vi "PulseDetect80AndSwitch160_10_HostTest.vi"(6 "Switch for":i32=6, 8 "Fill from last":i32=6, 9 "Laser bits in":bool[](array[boolean])=[FALSE, FALSE, FALSE, FALSE, FALSE, FALSE, FALSE, FALSE, FALSE, FALSE], 10 "Last area in":bool=TRUE, 11 "Last laser bit in":bool) -> (0 "Fill after last":i32=6, 1 "Area array out":bool[](array[boolean]), 2 "New last area out":bool, 3 "New last laser bit out":bool)   [LabVIEW 2012]
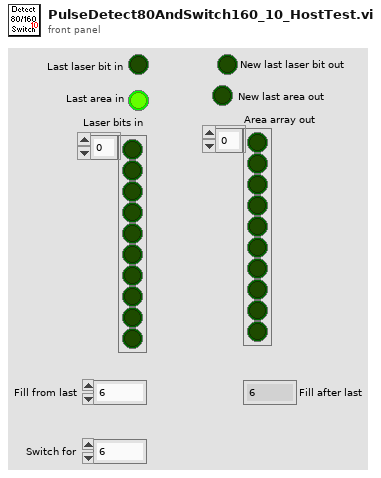
[diagram p1: front panel]
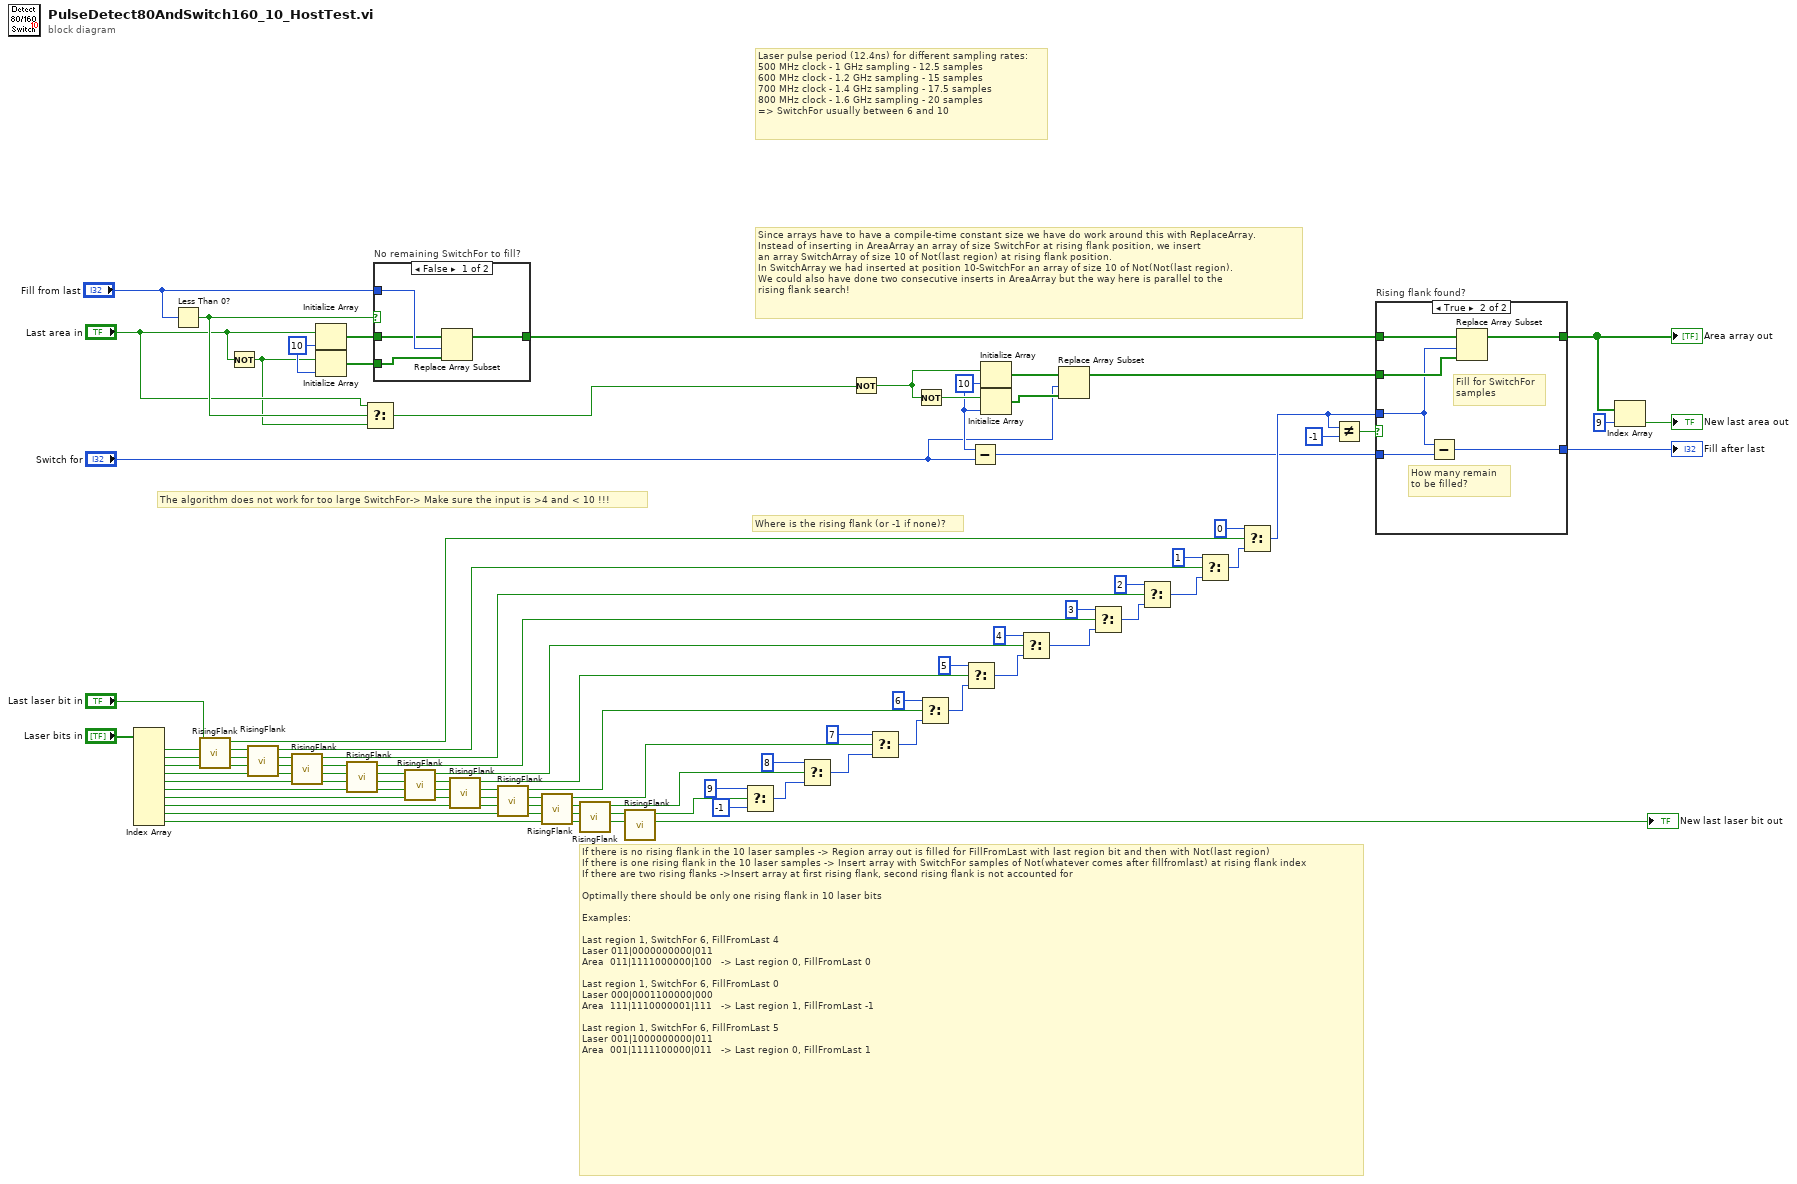
[diagram p0: block diagram]
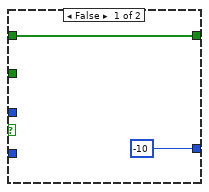
[diagram p3: hidden frame]
diagram:
  w7 = 10 ("dimension size")
  w15 = 10 ("dimension size")
  # "Since arrays have to have a compile-time constant size we have do work around this with ReplaceArray.\nInstead of inserting in AreaArray an array of size SwitchFor at rising flank position, we insert \nan array SwitchArray of size 10 of Not(last region) at rising flank position.\nIn SwitchArray we had inserted at position 10-SwitchFor an array of size 10 of Not(Not(last region).\nWe could also have done two consecutive inserts in AreaArray but the way here is parallel to the \nrising flank search!"
  # "The algorithm does not work for too large SwitchFor-> Make sure the input is >4 and < 10 !!!"
  # "Where is the rising flank (or -1 if none)?"
  # "Laser pulse period (12.4ns) for different sampling rates:\n500 MHz clock - 1 GHz sampling - 12.5 samples\n600 MHz clock - 1.2 GHz sampling - 15 samples\n700 MHz clock - 1.4 GHz sampling - 17.5 samples\n800 MHz clock - 1.6 GHz sampling - 20 samples \n=> SwitchFor usually between 6 and 10"
  # "If there is no rising flank in the 10 laser samples -> Region array out is filled for FillFromLast with last region bit and then with Not(last region)\nIf there is one rising flank in the 10 laser samples -> Insert array with SwitchFor samples of Not(whatever comes after fillfromlast) at rising flank index\nIf there are two rising flanks ->Insert array at first rising flank, second rising flank is not accounted for\n\nOptimally there should be only one rising flank in 10 laser bits\n\nExamples:\n\nLast region 1, SwitchFor 6, FillFromLast 4\nLaser 011|0000000000|011\nArea  011|1111000000|100   -> Last region 0, FillFromLast 0\n\nLast region 1, SwitchFor 6, FillFromLast 0\nLaser 000|0001100000|000\nArea  111|1110000001|111   -> Last region 1, FillFromLast -1\n\nLast region 1, SwitchFor 6, FillFromLast 5\nLaser 001|1000000000|011\nArea  001|1111100000|011   -> Last region 0, FillFromLast 1"
  n1 = Index Array(array="Laser bits in") -> (element #1=w64:bool, element #2=w63:bool, element #3=w62:bool, element #4=w61:bool, element #5=w60:bool, element #6=w59:bool, element #7=w58:bool, element #8=w57:bool, element #9=w56:bool, element #10=w38:bool)  [unwired: 10 in]
  "New last laser bit out" <- w38
  n2 = Less Than 0?(x="Fill from last") -> (x < 0?=w4:bool)
  n3 = call "RisingFlank.vi"("2nd sample"=w64, "1st sample"="Last laser bit in") -> ("Rising flank?"=w55:bool)  [unwired: 7 in]
  n4 = Not(x="Last area in") -> (.not. x?=w2:bool)
  n5 = call "RisingFlank.vi"("2nd sample"=w63, "1st sample"=w64) -> ("Rising flank?"=w53:bool)  [unwired: 7 in]
  n6 = call "RisingFlank.vi"("2nd sample"=w62, "1st sample"=w63) -> ("Rising flank?"=w51:bool)  [unwired: 7 in]
  n7 = Initialize Array("Last area in", w15) -> (w16:bool[])
  n8 = Initialize Array(w2, w15) -> (w14:bool[])
  n9 = call "RisingFlank.vi"("2nd sample"=w61, "1st sample"=w62) -> ("Rising flank?"=w36:bool)  [unwired: 7 in]
  n10 = Select(t="Last area in", s=w4, f=w2) -> (s? t:f=w1:bool)
  n11 = case "No remaining SwitchFor to fill?" shown="False" w4 {
    tunnel: [w67 w71] -> w13
    tunnel: "Fill from last" -> [w70 _]
    tunnel: w16 -> [w69 w71]
    tunnel: w14 -> [w68 _]
    frame False {
      n12 = Replace Array Subset(array=w69, new element=w68, index=w70) -> (w67:bool[])
    }
    frame True {
    }
  }
  n13 = call "RisingFlank.vi"("2nd sample"=w60, "1st sample"=w61) -> ("Rising flank?"=w49:bool)  [unwired: 7 in]
  n14 = call "RisingFlank.vi"("2nd sample"=w59, "1st sample"=w60) -> ("Rising flank?"=w47:bool)  [unwired: 7 in]
  n15 = call "RisingFlank.vi"("2nd sample"=w58, "1st sample"=w59) -> ("Rising flank?"=w45:bool)  [unwired: 7 in]
  n16 = call "RisingFlank.vi"("2nd sample"=w57, "1st sample"=w58) -> ("Rising flank?"=w43:bool)  [unwired: 7 in]
  n17 = call "RisingFlank.vi"("2nd sample"=w56, "1st sample"=w57) -> ("Rising flank?"=w41:bool)  [unwired: 7 in]
  n18 = call "RisingFlank.vi"("2nd sample"=w38, "1st sample"=w56) -> ("Rising flank?"=w39:bool)  [unwired: 7 in]
  n19 = Select(t=9, s=w39, f=-1) -> (s? t:f=w28:i32)
  n20 = Select(t=8, s=w41, f=w28) -> (s? t:f=w27:i32)
  n21 = Not(x=w1) -> (.not. x?=w11:bool)
  n22 = Select(t=7, s=w43, f=w27) -> (s? t:f=w26:i32)
  n23 = Not(x=w11) -> (.not. x?=w9:bool)
  n24 = Select(t=6, s=w45, f=w26) -> (s? t:f=w25:i32)
  n25 = Select(t=5, s=w47, f=w25) -> (s? t:f=w24:i32)
  n26 = Subtract(x=w7, y="Switch for") -> (x-y=w6:i32)
  n27 = Initialize Array(w11, w7) -> (w12:bool[])
  n28 = Initialize Array(w9, w7) -> (w8:bool[])
  n29 = Select(t=4, s=w49, f=w24) -> (s? t:f=w23:i32)
  n30 = Replace Array Subset(array=w12, new element=w8, index="Switch for") -> (w10:bool[])
  n31 = Select(t=3, s=w36, f=w23) -> (s? t:f=w22:i32)
  n32 = Select(t=2, s=w51, f=w22) -> (s? t:f=w21:i32)
  n33 = Select(t=1, s=w53, f=w21) -> (s? t:f=w20:i32)
  n34 = Select(t=0, s=w55, f=w20) -> (s? t:f=w19:i32)
  n35 = Not Equal?(x=w19, y=-1) -> (x != y?=w34:bool)
  n36 = case "Rising flank found?" shown="True" w34 {
    tunnel: w13 -> [w73 w79]
    tunnel: w10 -> [_ w78]
    tunnel: w19 -> [_ w76]
    tunnel: [w73 w77] -> w32
    tunnel: [-10 w75] -> w18
    tunnel: w6 -> [_ w74]
    frame False {
    }
    frame True {
      # "Fill for SwitchFor\nsamples"
      # "How many remain\nto be filled?"
      n37 = Subtract(x=w76, y=w74) -> (x-y=w75:i32)
      n38 = Replace Array Subset(array=w79, new element=w78, index=w76) -> (w77:bool[])
    }
  }
  "Area array out" <- w32
  "Fill after last" <- w18
  n39 = Index Array(array=w32, index=9) -> (element=→"New last area out":bool)
